vi "Update Coins.vi"(8 "error in (no error)":errorcluster, 10 "Credito Update":dbl, 11 "MXN Actor in":refnum<class "MXN Actor.lvclass">) -> (0 "error out":errorcluster, 3 "MXN Actor out":refnum<class "MXN Actor.lvclass">)   [LabVIEW 2020, in "MXN Actor.lvlib" / "MXN Actor.lvclass"]
uses:
  MXN Actor.lvclass
  MXN Actor.lvclass/MXN Actor.ctl
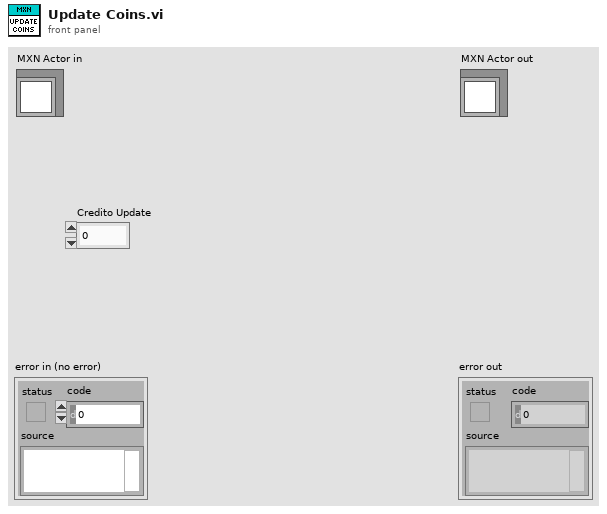
[diagram p1: front panel]
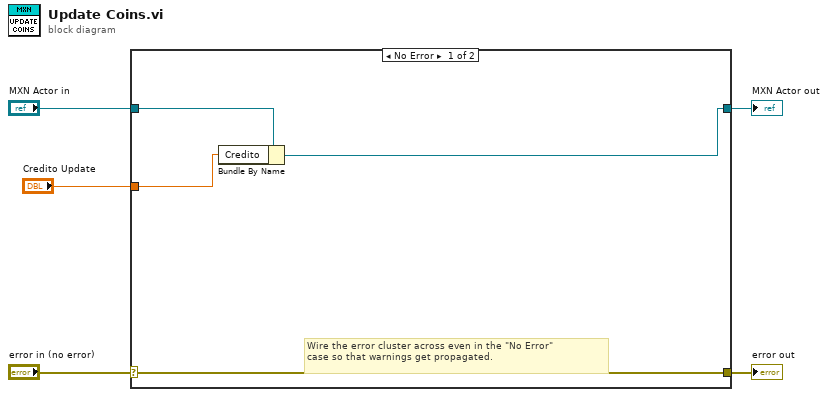
[diagram p0: block diagram]
diagram:
  n1 = case shown="No Error" "error in (no error)" {
    selector: "error in (no error)" -> [w9 w11]
    tunnel: [w9 w11] -> w4
    tunnel: [w6 w10] -> w2
    tunnel: "MXN Actor in" -> [w8 w10]
    tunnel: "Credito Update" -> [w7 _]
    frame No Error {
      # "Wire the error cluster across even in the \"No Error\"\ncase so that warnings get propagated."
      n2 = Bundle By Name(cluster=w8, "Credito"=w7) -> (w6:refnum<class "MXN Actor.lvclass">)
    }
    frame Error {
    }
  }
  "error out" <- w4
  "MXN Actor out" <- w2
